vi "PH_Sound.PC Play Single Tone.vi"(0 "VI in":refnum<vi>, 2 "Tone":dbl, 3 "Length [ms]":i32, 5 "error in (no error)":errorcluster) -> (14 "VI out":refnum<vi>, 19 "error out":errorcluster)   [LabVIEW 2014, in "PH_Sound.lvlib"]
uses:
  PH_Sound.lvlib
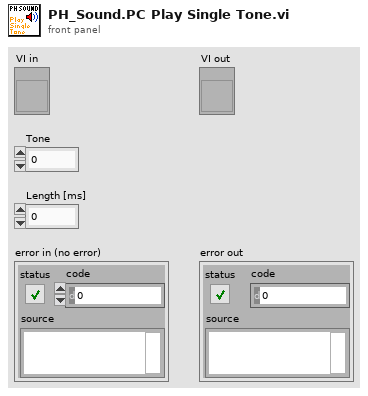
[diagram p1: front panel]
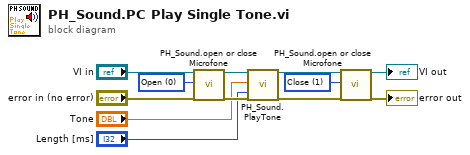
[diagram p0: block diagram]
diagram:
  w5 = u16 1 items=["Open", "Close"] ("Action")
  w2 = u16 0 items=["Open", "Close"] ("Action")
  n1 = call "PH_Sound.open or close Microfone.vi"("i ref in"="VI in", "Action"=w2, "error in (no error)"="error in (no error)") -> ("i ref out"=w11:refnum<vi>, "error out"=w10:errorcluster)  [unwired: 15 in]
  n2 = call "PH_Sound.PlayTone.vi"("VI in"=w11, "tone"="Tone", "length [ms]"="Length [ms]", "error in"=w10) -> ("VI out"=w12:refnum<vi>, "error out"=w6:errorcluster)  [unwired: 14 in]
  n3 = call "PH_Sound.open or close Microfone.vi"("i ref in"=w12, "Action"=w5, "error in (no error)"=w6) -> ("i ref out"=→"VI out":refnum<vi>, "error out"=→"error out":errorcluster)  [unwired: 15 in]
